vi "Create ClassName ComboBox.vi"() -> ()   [LabVIEW 2011]
uses:
  Application.lvlib
panel:
  out "ClassName":string(combo)
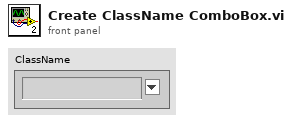
[diagram p1: front panel]
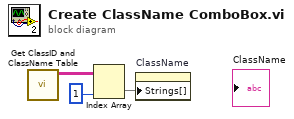
[diagram p0: block diagram]
diagram:
  n1 = call "Get ClassID and ClassName Table.vi"() -> ("ClassID and ClassName"=w3:string[][])  [unwired: 10 in, 1 out]
  n2 = Index Array(array=w3, index (col)=1 ("禁用的索引 (列)")) -> (element=w1:string[])  [unwired: 1 in]
  n3 = property on="ClassName" class="CmbBox"("Strings[]"=w1) -> ()  [unwired: 2 in, 2 out]
